vi "Main_UI.vi"() -> ()   [LabVIEW 2012]
uses:
  Donate.ctl
  PortFolio-Provider.ctl
  UI Refs.ctl
  Actions.ctl
  PortFolio/Portfolio.lvclass/Portfolio.ctl
  <vilib>/Utility/miscctls.llb/LVRowAndColumnTypeDef.ctl
  PortFolio/Find_Exchanges.ctl
  PortFolio/Portfolio.lvclass
  Operations/Operations.lvclass
  Exchanges/Exchanges.lvclass
panel:
  in  "Donate":T1
  out "calc Done ?":bool
  out "Current Portfolio Path":path
  out "Version":string="XLPortFolio"
  out "Config File Path":path
  out "Libelles File Path":path
  in  "Search Stock":bool
  in  "Help":bool
  in  "Save":bool
  in  "Print":bool
  in  "Collapse Left":bool
  in  "TabControl":T2(tab)
  out "Performance sur 1an :":sgl format="%.2f%"
  out "% cash":sgl format="%.2f%"
  out "% investi":sgl format="%.2f%"
  out "Montant investi :":sgl format="%.2f€"
  out "Performance Totale :":sgl format="%.2f%"
  out "Investissement total :":sgl format="%.2f€"
  out "Solde Liquidation :":sgl format="%.2f€"
  out "Valeur veille :":sgl format="%.2f€"
  out "Solde espèces :":sgl format="%.2f€"
  out "Evaluation totale :":dbl format="%.2f€"
  in  "Portefeuille":i32(listbox)
  in  "Mettre a jour les cours":bool
  in  "Delete Exch":bool
  in  "Edit Exch":bool
  in  "Add Exch":bool
  in  "Exchanges":i32[](listbox)
  in  "Operations":i32[](listbox)
  in  "Add OP":bool
  in  "Edit OP":bool
  in  "Delete OP":bool
  out "Waveform Graph":waveform(dbl)[](graph)
  in  "Update Hist":bool
  out "Tarifs":waveform(dbl)[](graph) caption="Tarifs des portails Bourses 2017 (en % de Frais)"
  in  "Provider":T3
  out "Table Control 2":string[][](table)=[["12/31/1903 6:00:00 PM", "-0.052"], ["12/31/1903 6:00:00 PM", "-0.133"], ["12/31/1903 6:00:00 PM", "0.097"], ["12/31/1903 6:00:00 PM", "0.043"], ["12/31/1903 6:00:00 PM", "0.408"], ["12/31/1903 6:00:00 PM", "0.144"], ["12/31/1903 6:00:00 PM", "0.183"], ["12/31/1903 6:00:00 PM", "0.589"], ["12/31/1903 6:00:00 PM", "0.287"], ["12/31/1903 6:00:00 PM", "0.424"], ["12/31/1903 6:00:00 PM", "0.399"], ["12/31/1903 6:00:00 PM", "0.495"], ["12/31/1903 6:00:00 PM", "0.848"], ["12/31/1903 6:00:00 PM", "0.550"], ["12/31/1903 6:00:00 PM", "0.762"], ["12/31/1903 6:00:00 PM", "0.686"], ["12/31/1903 6:00:00 PM", "0.766"], ["12/31/1903 6:00:00 PM", "0.760"], ["12/31/1903 6:00:00 PM", "0.913"], ["12/31/1903 6:00:00 PM", "0.929"], ["12/31/1903 6:00:00 PM", "0.800"], ["12/31/1903 6:00:00 PM", "0.958"], ["12/31/1903 6:00:00 PM", "1.034"], ["12/31/1903 6:00:00 PM", "1.183"], ["12/31/1903 6:00:00 PM", "1.132"], ["12/31/1903 6:00:00 PM", "1.155"], ["12/31/1903 6:00:00 PM", "0.931"], ["12/31/1903 6:00:00 PM", "1.036"], ["12/31/1903 6:00:00 PM", "0.780"], ["12/31/1903 6:00:00 PM", "0.999"], ["12/31/1903 6:00:00 PM", "0.907"], ["12/31/1903 6:00:00 PM", "0.915"], ["12/31/1903 6:00:00 PM", "0.726"], ["12/31/1903 6:00:00 PM", "0.758"], ["12/31/1903 6:00:00 PM", "0.769"], ["12/31/1903 6:00:00 PM", "0.879"], ["12/31/1903 6:00:00 PM", "0.573"], ["12/31/1903 6:00:00 PM", "0.830"], ["12/31/1903 6:00:00 PM", "0.796"], ["12/31/1903 6:00:00 PM", "0.546"], ["12/31/1903 6:00:00 PM", "0.413"], ["12/31/1903 6:00:00 PM", "0.602"], ["12/31/1903 6:00:00 PM", "0.547"], ["12/31/1903 6:00:00 PM", "0.573"], ["12/31/1903 6:00:00 PM", "0.326"], ["12/31/1903 6:00:00 PM", "0.432"], ["12/31/1903 6:00:00 PM", "0.132"], ["12/31/1903 6:00:00 PM", "0.157"], ["12/31/1903 6:00:00 PM", "0.194"], ["12/31/1903 6:00:00 PM", "-0.046"], ["12/31/1903 6:00:00 PM", "-0.219"], ["12/31/1903 6:00:00 PM", "-0.209"], ["12/31/1903 6:00:00 PM", "0.007"], ["12/31/1903 6:00:00 PM", "-0.095"], ["12/31/1903 6:00:00 PM", "-0.433"], ["12/31/1903 6:00:00 PM", "-0.258"], ["12/31/1903 6:00:00 PM", "-0.357"], ["12/31/1903 6:00:00 PM", "-0.548"], ["12/31/1903 6:00:00 PM", "-0.712"], ["12/31/1903 6:00:00 PM", "-0.686"], ["12/31/1903 6:00:00 PM", "-0.709"], ["12/31/1903 6:00:00 PM", "-0.790"], ["12/31/1903 6:00:00 PM", "-0.635"], ["12/31/1903 6:00:00 PM", "-0.851"], ["12/31/1903 6:00:00 PM", "-0.953"], ["12/31/1903 6:00:00 PM", "-0.886"], ["12/31/1903 6:00:00 PM", "-0.810"], ["12/31/1903 6:00:00 PM", "-0.966"], ["12/31/1903 6:00:00 PM", "-0.804"], ["12/31/1903 6:00:00 PM", "-1.056"], ["12/31/1903 6:00:00 PM", "-1.070"], ["12/31/1903 6:00:00 PM", "-1.027"], ["12/31/1903 6:00:00 PM", "-0.951"], ["12/31/1903 6:00:00 PM", "-0.862"], ["12/31/1903 6:00:00 PM", "-0.844"], ["12/31/1903 6:00:00 PM", "-1.160"], ["12/31/1903 6:00:00 PM", "-0.880"], ["12/31/1903 6:00:00 PM", "-0.949"], ["12/31/1903 6:00:00 PM", "-1.011"], ["12/31/1903 6:00:00 PM", "-0.802"], ["12/31/1903 6:00:00 PM", "-0.767"], ["12/31/1903 6:00:00 PM", "-0.893"], ["12/31/1903 6:00:00 PM", "-0.788"], ["12/31/1903 6:00:00 PM", "-0.897"], ["12/31/1903 6:00:00 PM", "-0.635"], ["12/31/1903 6:00:00 PM", "-0.592"], ["12/31/1903 6:00:00 PM", "-0.541"], ["12/31/1903 6:00:00 PM", "-0.574"], ["12/31/1903 6:00:00 PM", "-0.511"], ["12/31/1903 6:00:00 PM", "-0.541"], ["12/31/1903 6:00:00 PM", "-0.648"], ["12/31/1903 6:00:00 PM", "-0.499"], ["12/31/1903 6:00:00 PM", "-0.624"], ["12/31/1903 6:00:00 PM", "-0.271"], ["12/31/1903 6:00:00 PM", "-0.120"], ["12/31/1903 6:00:00 PM", "-0.199"], ["12/31/1903 6:00:00 PM", "-0.335"], ["12/31/1903 6:00:00 PM", "-0.056"], ["12/31/1903 6:00:00 PM", "-0.195"], ["12/31/1903 6:00:00 PM", "-0.065"]]
  in  "Collapse Right":bool
  out "Table Control":string[][](table)=[["12/31/1903 6:00:00 PM", "-0.052"], ["12/31/1903 6:00:00 PM", "-0.133"], ["12/31/1903 6:00:00 PM", "0.097"], ["12/31/1903 6:00:00 PM", "0.043"], ["12/31/1903 6:00:00 PM", "0.408"], ["12/31/1903 6:00:00 PM", "0.144"], ["12/31/1903 6:00:00 PM", "0.183"], ["12/31/1903 6:00:00 PM", "0.589"], ["12/31/1903 6:00:00 PM", "0.287"], ["12/31/1903 6:00:00 PM", "0.424"], ["12/31/1903 6:00:00 PM", "0.399"], ["12/31/1903 6:00:00 PM", "0.495"], ["12/31/1903 6:00:00 PM", "0.848"], ["12/31/1903 6:00:00 PM", "0.550"], ["12/31/1903 6:00:00 PM", "0.762"], ["12/31/1903 6:00:00 PM", "0.686"], ["12/31/1903 6:00:00 PM", "0.766"], ["12/31/1903 6:00:00 PM", "0.760"], ["12/31/1903 6:00:00 PM", "0.913"], ["12/31/1903 6:00:00 PM", "0.929"], ["12/31/1903 6:00:00 PM", "0.800"], ["12/31/1903 6:00:00 PM", "0.958"], ["12/31/1903 6:00:00 PM", "1.034"], ["12/31/1903 6:00:00 PM", "1.183"], ["12/31/1903 6:00:00 PM", "1.132"], ["12/31/1903 6:00:00 PM", "1.155"], ["12/31/1903 6:00:00 PM", "0.931"], ["12/31/1903 6:00:00 PM", "1.036"], ["12/31/1903 6:00:00 PM", "0.780"], ["12/31/1903 6:00:00 PM", "0.999"], ["12/31/1903 6:00:00 PM", "0.907"], ["12/31/1903 6:00:00 PM", "0.915"], ["12/31/1903 6:00:00 PM", "0.726"], ["12/31/1903 6:00:00 PM", "0.758"], ["12/31/1903 6:00:00 PM", "0.769"], ["12/31/1903 6:00:00 PM", "0.879"], ["12/31/1903 6:00:00 PM", "0.573"], ["12/31/1903 6:00:00 PM", "0.830"], ["12/31/1903 6:00:00 PM", "0.796"], ["12/31/1903 6:00:00 PM", "0.546"], ["12/31/1903 6:00:00 PM", "0.413"], ["12/31/1903 6:00:00 PM", "0.602"], ["12/31/1903 6:00:00 PM", "0.547"], ["12/31/1903 6:00:00 PM", "0.573"], ["12/31/1903 6:00:00 PM", "0.326"], ["12/31/1903 6:00:00 PM", "0.432"], ["12/31/1903 6:00:00 PM", "0.132"], ["12/31/1903 6:00:00 PM", "0.157"], ["12/31/1903 6:00:00 PM", "0.194"], ["12/31/1903 6:00:00 PM", "-0.046"], ["12/31/1903 6:00:00 PM", "-0.219"], ["12/31/1903 6:00:00 PM", "-0.209"], ["12/31/1903 6:00:00 PM", "0.007"], ["12/31/1903 6:00:00 PM", "-0.095"], ["12/31/1903 6:00:00 PM", "-0.433"], ["12/31/1903 6:00:00 PM", "-0.258"], ["12/31/1903 6:00:00 PM", "-0.357"], ["12/31/1903 6:00:00 PM", "-0.548"], ["12/31/1903 6:00:00 PM", "-0.712"], ["12/31/1903 6:00:00 PM", "-0.686"], ["12/31/1903 6:00:00 PM", "-0.709"], ["12/31/1903 6:00:00 PM", "-0.790"], ["12/31/1903 6:00:00 PM", "-0.635"], ["12/31/1903 6:00:00 PM", "-0.851"], ["12/31/1903 6:00:00 PM", "-0.953"], ["12/31/1903 6:00:00 PM", "-0.886"], ["12/31/1903 6:00:00 PM", "-0.810"], ["12/31/1903 6:00:00 PM", "-0.966"], ["12/31/1903 6:00:00 PM", "-0.804"], ["12/31/1903 6:00:00 PM", "-1.056"], ["12/31/1903 6:00:00 PM", "-1.070"], ["12/31/1903 6:00:00 PM", "-1.027"], ["12/31/1903 6:00:00 PM", "-0.951"], ["12/31/1903 6:00:00 PM", "-0.862"], ["12/31/1903 6:00:00 PM", "-0.844"], ["12/31/1903 6:00:00 PM", "-1.160"], ["12/31/1903 6:00:00 PM", "-0.880"], ["12/31/1903 6:00:00 PM", "-0.949"], ["12/31/1903 6:00:00 PM", "-1.011"], ["12/31/1903 6:00:00 PM", "-0.802"], ["12/31/1903 6:00:00 PM", "-0.767"], ["12/31/1903 6:00:00 PM", "-0.893"], ["12/31/1903 6:00:00 PM", "-0.788"], ["12/31/1903 6:00:00 PM", "-0.897"], ["12/31/1903 6:00:00 PM", "-0.635"], ["12/31/1903 6:00:00 PM", "-0.592"], ["12/31/1903 6:00:00 PM", "-0.541"], ["12/31/1903 6:00:00 PM", "-0.574"], ["12/31/1903 6:00:00 PM", "-0.511"], ["12/31/1903 6:00:00 PM", "-0.541"], ["12/31/1903 6:00:00 PM", "-0.648"], ["12/31/1903 6:00:00 PM", "-0.499"], ["12/31/1903 6:00:00 PM", "-0.624"], ["12/31/1903 6:00:00 PM", "-0.271"], ["12/31/1903 6:00:00 PM", "-0.120"], ["12/31/1903 6:00:00 PM", "-0.199"], ["12/31/1903 6:00:00 PM", "-0.335"], ["12/31/1903 6:00:00 PM", "-0.056"], ["12/31/1903 6:00:00 PM", "-0.195"], ["12/31/1903 6:00:00 PM", "-0.065"]]
  in  "Cancel":bool
  out "Progress Bar":u8(slide) scale=0.0..100.0
  out "Status Bar Text":string="This is the status bar!"
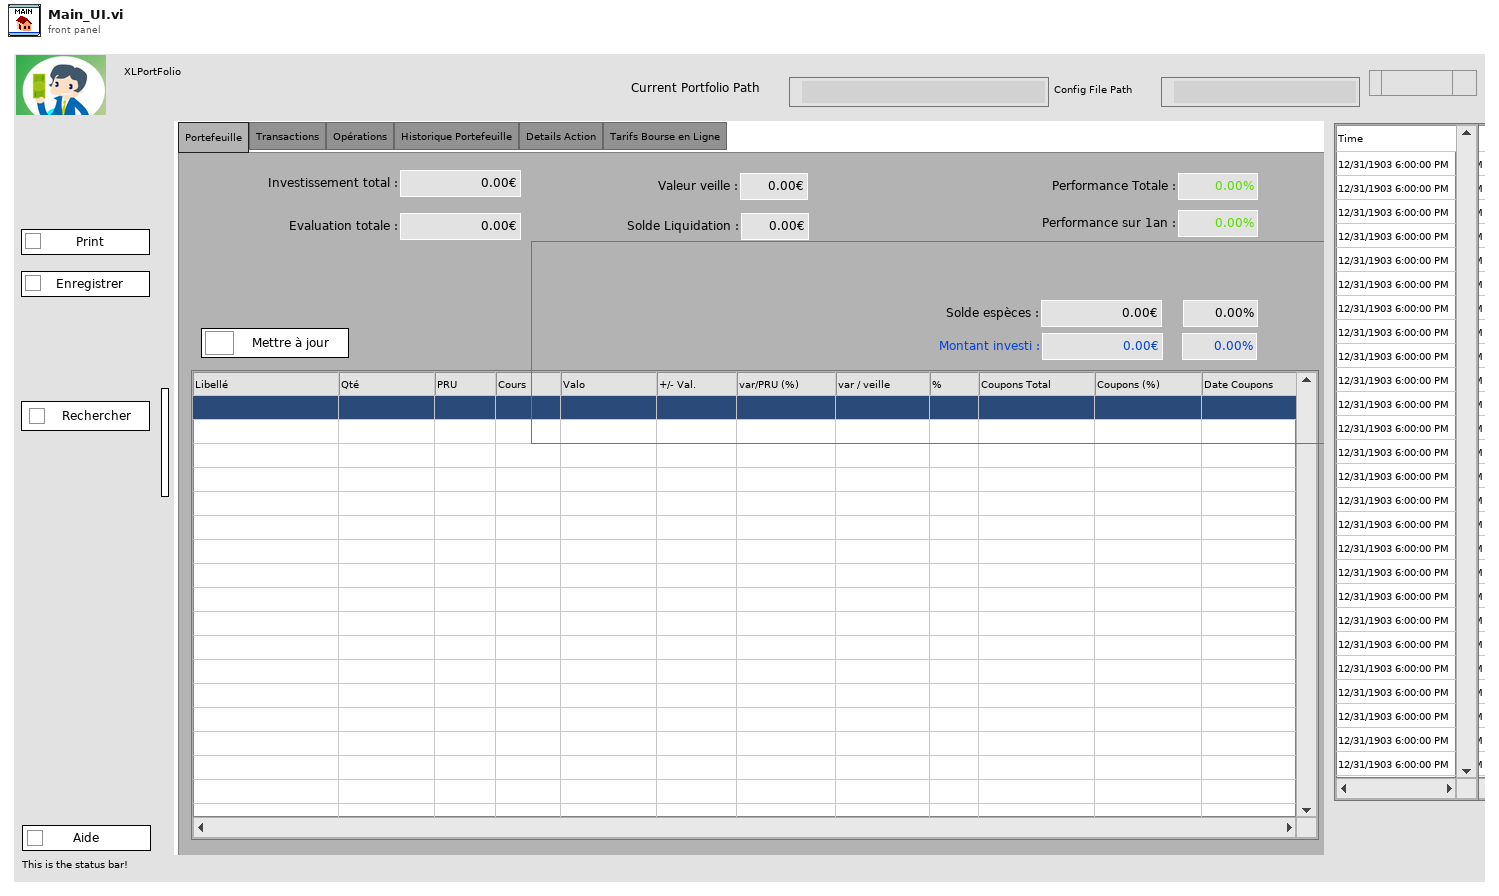
[diagram p1: front panel]
types:
  T1 = typedef "Donate.ctl" = bool
  T2 = enum32{"Portefeuille", "Transactions", "Opérations", "Historique Portefeuille", "Details Action", "Tarifs Bourse en Ligne"}
  T3 = typedef "PortFolio-Provider.ctl" = enum16{"Bourse Direct", "Binck classique", "Boursorama Découverte", "Boursorama Classique", "Boursorama Trader", "Boursorama Ultimate Trader", "IG Actions Euro"}
  T4 = cluster{"Select Printer":string, "Limit number of pages":dbl, "Filename":path, "Prompt for file path":bool, "When saving multiple files":enum32{"Radio Selection 1", "Radio Selection 2"}}
  T5 = enum32{"Portefeuille", "Transactions", "Opérations", "Historique Portefeuille"}
  T6 = typedef "UI Refs.ctl" = cluster{"Cancel Button Ref":refnum<vi>, "Status Bar Text Ref":refnum<vi>, "Progress Bar Ref":refnum<vi>, "This VI":refnum<vi>}
  T7 = typedef "Actions.ctl" = enum16{"Calc", "Calc History", "Test Progress Bar", "Help", "Panel Resize", "Print", "Donate", "Acquire", "Save Portfolio", "New Portfolio", "Open Portfolio", "Add Operation", "Edit Operation", "Delete Operation", "Add Exchange", "Edit Exchange", "Update Operations", "Update Exchanges", "Delete Exchange", "Display tarif", "Update PFLine ToolStrip"}
  T8 = enum8{"Enabled", "Disabled", "Disabled and Grayed Out"}
  T9 = cluster{"FileVersion":string, "FileMajorPart":i32, "FileMinorPart":i32, "FileBuildPart":i32, "FilePrivatePart":i32, "Language":string, "LegalCopyright":string, "FileDescription":string, "CompanyName":string, "ProductName":string, "InternalName":string}
  T10 = typedef "LVRowAndColumnTypeDef.ctl" = cluster{"Row":i32, "Column":i32}
  T11 = typedef "Find_Exchanges.ctl" = enum16{"Find_From_Label", "Find_From_ISIN"}
  T12 = typedef "Portfolio Parameters.ctl" = cluster{"Date":timestamp, "Name":string, "Cash":dbl, "Total":dbl, "Investissements":dbl, "Performance Totale (en %)":dbl, "Performance sur 1 an (en %)":dbl}
  T13 = typedef "Operation Parameters.ctl" = cluster{"Date":timestamp, "Operation Type":T14, "Amount":dbl, "Comment":string, "Currency":T15}
  T14 = typedef "Operation Type Enum.ctl" = enum16{"Coupons", "Dépot", "Retrait", "Intérêts", "Taxe"}
  T15 = typedef "Currencies.ctl" = enum16{"Euro", "Dollar", "Yen", "RIM", "CHF"}
  T16 = typedef "Exchange Parameters.ctl" = cluster{"Date":timestamp, "Exchange Type":T17, "ISIN":string, "Label":string, "Price":dbl, "Qty":dbl, "Currency":T15, "Tax":dbl, "Comment":string, "PRU":dbl}
  T17 = typedef "Exchange.lvclass/Exchange Type Enum.ctl" = enum16{"ACHAT", "VENTE"}
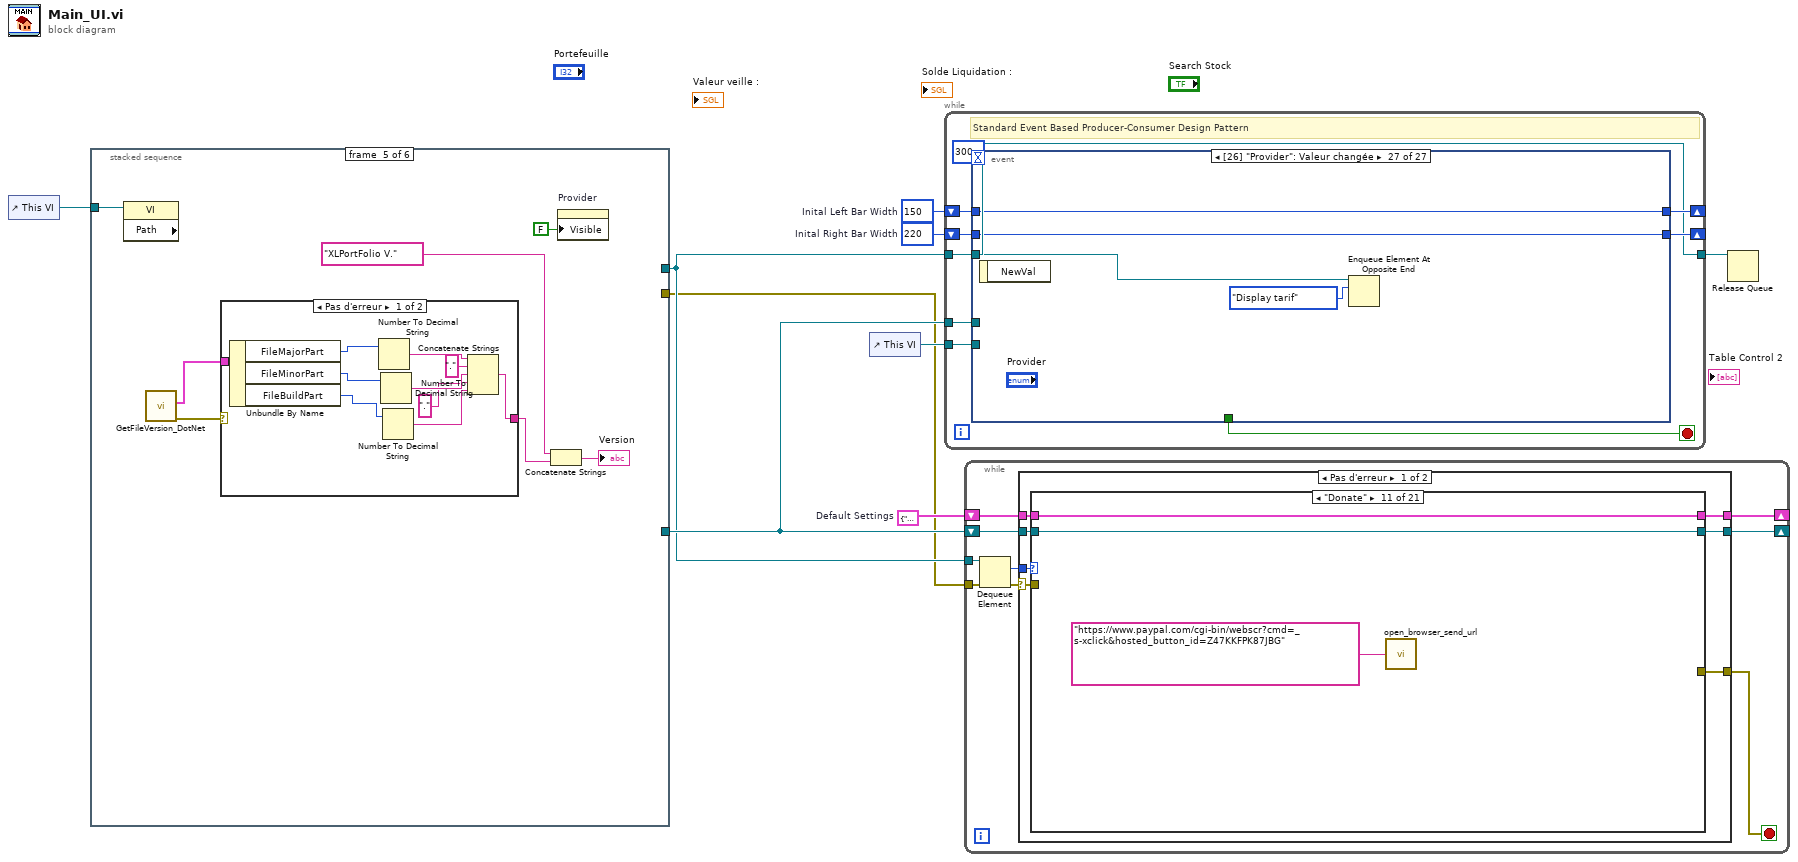
[diagram p0: block diagram]
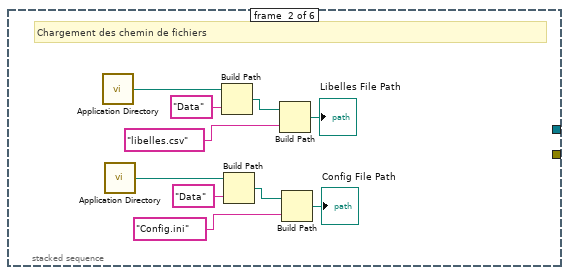
[diagram p3: hidden frame]
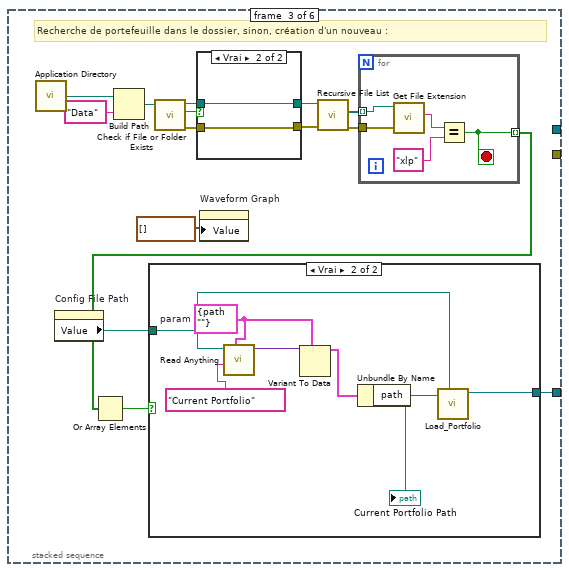
[diagram p4: hidden frame]
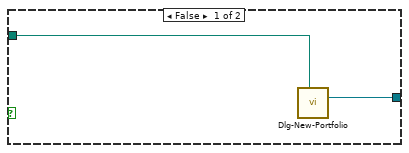
[diagram p5: hidden frame]
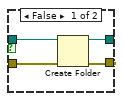
[diagram p6: hidden frame]
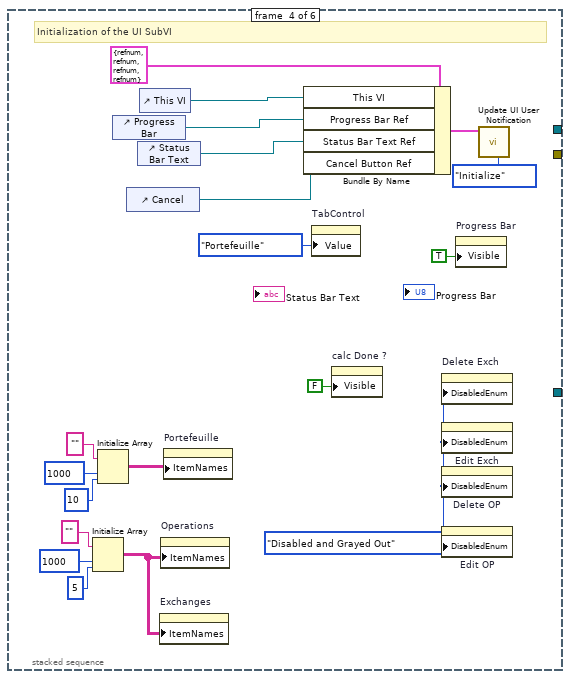
[diagram p7: hidden frame]
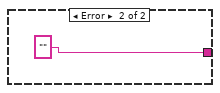
[diagram p8: hidden frame]
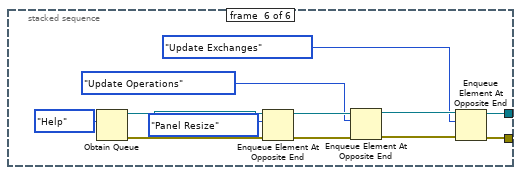
[diagram p9: hidden frame]
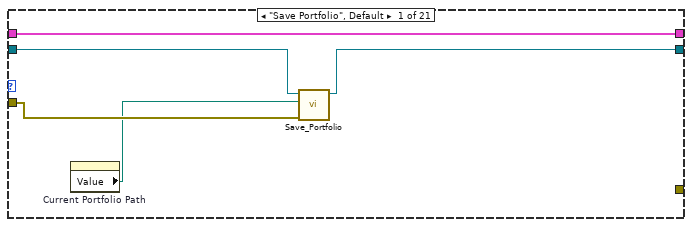
[diagram p10: hidden frame]
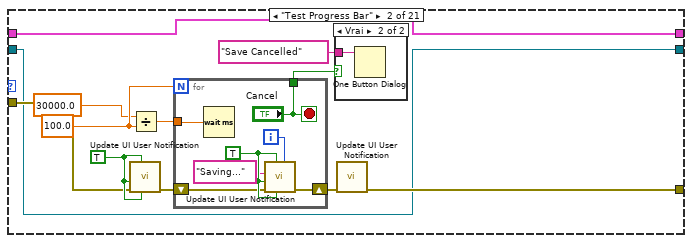
[diagram p11: hidden frame]
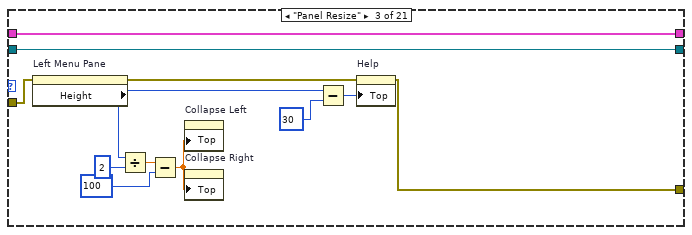
[diagram p13: hidden frame]
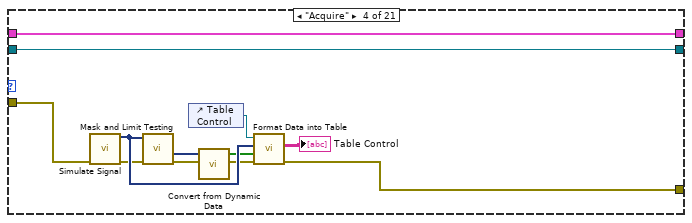
[diagram p14: hidden frame]
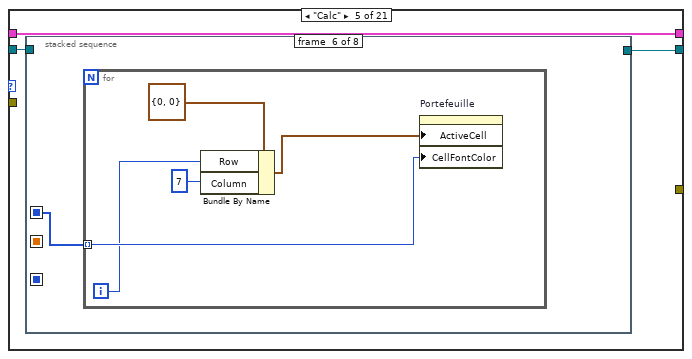
[diagram p15: hidden frame]
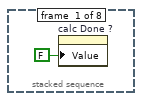
[diagram p16: hidden frame]
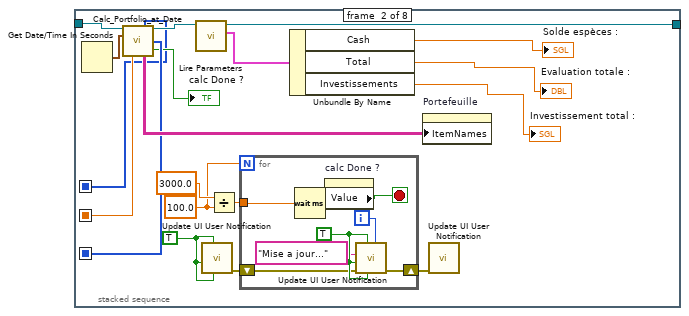
[diagram p17: hidden frame]
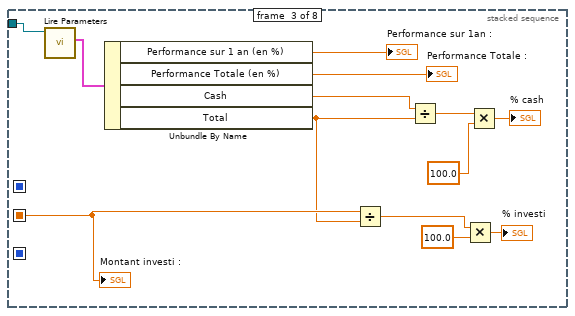
[diagram p18: hidden frame]
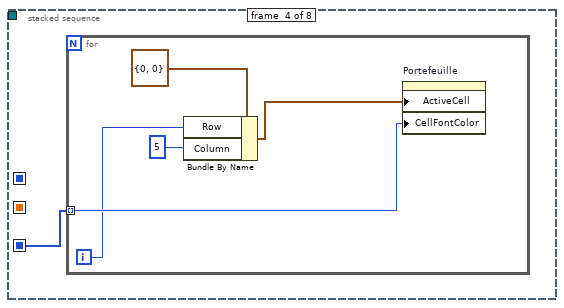
[diagram p19: hidden frame]
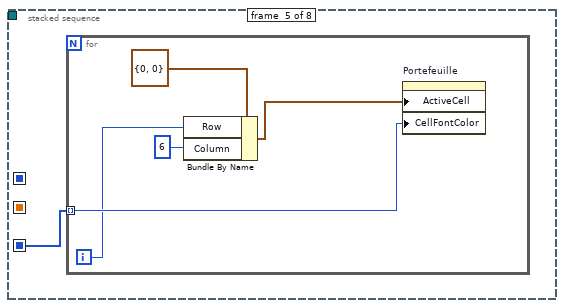
[diagram p20: hidden frame]
diagram:
  w5 = T4 {"Select Printer"="Lab Printer 1", "Limit number of pages"=3.0, "Filename"=path "", "Prompt for file path"=FALSE, "When saving multiple files"=enum."Radio Selection 1"}  # Default Settings
  w8 = 220  # Inital Right Bar Width
  w9 = 150  # Inital Left Bar Width
  n1 = control-ref of="This VI"() -> (w1:refnum<vi>)
  n2 = stacked-sequence {
    tunnel: [_ _ _ _ _ w94] -> w2
    tunnel: [_ _ w34 _ _ _] -> w4
    tunnel: [_ _ _ _ _ w97] -> w3
    tunnel: w1 -> [_ _ _ _ w77 _]
    frame #0 {
    }
    frame #1 {
      # "Chargement des chemin de fichiers"
      n3 = call <vilib>:"Application Directory.vi"() -> ("Application Directory"=w18:path)
      n4 = call <vilib>:"Application Directory.vi"() -> ("Application Directory"=w11:path)
      n5 = Build Path(base path=w18, name or relative path="Data" ("nom ou chemin relatif")) -> (appended path=w16:path)
      n6 = Build Path(base path=w11, name or relative path="Data" ("nom ou chemin relatif")) -> (appended path=w13:path)
      n7 = Build Path(base path=w16, name or relative path="libelles.csv" ("nom ou chemin relatif")) -> (appended path=→"Libelles File Path":path)
      n8 = Build Path(base path=w13, name or relative path="Config.ini" ("nom ou chemin relatif")) -> (appended path=→"Config File Path":path)
    }
    frame #2 {
      # "Recherche de portefeuille dans le dossier, sinon, création d'un nouveau :"
      n9 = call <vilib>:"Application Directory.vi"() -> ("Application Directory"=w33:path)
      n10 = property on="Config File Path" class="Chm"() -> ("Value"=w21:path)  [unwired: 2 in, 2 out]
      n11 = Build Path(base path=w33, name or relative path="Data" ("nom ou chemin relatif")) -> (appended path=w31:path)
      n12 = call <vilib>:"Check if File or Folder Exists.vi"("path"=w31) -> ("error out"=w28:errorcluster, "file or folder exists?"=w30:bool, "dup path"=w29:path)  [unwired: 8 in]
      n13 = case shown="Vrai" w30 {
        tunnel: w29 -> [w52 w53]
        tunnel: w28 -> [w51 w54]
        tunnel: [w50 w54] -> w26
        tunnel: [w49 w53] -> w27
        frame False {
          n14 = Create Folder(path (use dialog)=w52, error in=w51) -> (created path=w49:path, error out=w50:errorcluster)  [unwired: 1 in, 1 out]
        }
        frame True {
        }
      }
      n15 = property on="Waveform Graph" class="GraphWF (strict)"("Value"=waveform(dbl)[] [] ("Waveform Graph")) -> ()  [unwired: 2 in, 2 out]
      n16 = call <vilib>:"Recursive File List.vi"("error in (no error)"=w26, "Folder Path"=w27) -> ("error out"=w24:errorcluster, "All Files in Dir"=w25:path[])  [unwired: 5 in, 3 out]
      n17 = for {
        tunnel: w25 -> [w39] mode=indexing
        tunnel: w24 -> [w38]
        tunnel: [w35] -> w23 mode=indexing
        stop <- w35 stop-if-true
        n18 = call <vilib>:"Get File Extension.vi"("error in (no error)"=w38, "file"=w39) -> ("lowercase file extension"=w37:string)  [unwired: 6 in, 3 out]
        n19 = Equal?(x=w37, y="xlp") -> (x = y?=w35:bool)
      }
      n20 = Or Array Elements(Boolean array=w23) -> (logical OR=w22:bool)
      n21 = case shown="Vrai" w22 {
        tunnel: [w41 w46] -> w34
        tunnel: w21 -> [w40 w45]
        frame False {
          n22 = call "Dlg-New-Portfolio.vi"("Config File Path"=w40) -> ("Portfolio out"=w41:refnum<class "Portfolio.lvclass">)  [unwired: 8 in, 2 out]
        }
        frame True {
          w44 = cluster{"path":path} {"path"=path ""}  # param
          n23 = call "Read Anything.vi"("Type of Anything"=w44, "Section Name (Name of \"Type of Anything\")"="Current Portfolio" ("Section Name (Name of \"Anything\")"), "Path (dialog)"=w45) -> ("Anything"=w48:variant)  [unwired: 6 in, 2 out]
          n24 = Variant To Data(type=w44, Variant=w48) -> (data=w43:cluster{"path":path})  [unwired: 1 in, 1 out]
          n25 = Unbundle By Name(w43) -> ("path"=w42:path)
          "Current Portfolio Path" <- w42
          n26 = call "Load_Portfolio.vi"("Config File path"=w45, "path"=w42) -> ("Portfolio en sortie"=w46:refnum<class "Portfolio.lvclass">)  [unwired: 8 in, 1 out]
        }
      }
    }
    frame #3 {
      w57 = T8."Disabled and Grayed Out" ("Désactivé")
      # "Initialization of the UI SubVI"
      n27 = Initialize Array("", 1000, 5 ("taille de la dimension")) -> (w59:string[][])
      n28 = Initialize Array("", 1000, 10 ("taille de la dimension")) -> (w60:string[][])
      n29 = control-ref of="Progress Bar"() -> (w70:refnum<vi>)
      n30 = control-ref of="Cancel"() -> (w58:refnum<vi>)
      n31 = control-ref of="Status Bar Text"() -> (w69:refnum<vi>)
      n32 = control-ref of="This VI"() -> (w71:refnum<vi>)
      n33 = property on="Exchanges" class="ListeMCol (strict)"("ItemNames"=w59) -> ()  [unwired: 2 in, 2 out]
      n34 = property on="Operations" class="ListeMCol (strict)"("ItemNames"=w59) -> ()  [unwired: 2 in, 2 out]
      n35 = property on="Portefeuille" class="ListeMCol (strict)"("ItemNames"=w60) -> ()  [unwired: 2 in, 2 out]
      n36 = Bundle By Name(cluster=T6 {"Cancel Button Ref"=refnum, "Status Bar Text Ref"=refnum, "Progress Bar Ref"=refnum, "This VI"=refnum} ("UI Refs In"), "This VI"=w71, "Progress Bar Ref"=w70, "Status Bar Text Ref"=w69, "Cancel Button Ref"=w58) -> (w68:T6)
      n37 = property on="TabControl" class="Onglet (strict)"("Value"=T5."Portefeuille" ("TabControl")) -> ()  [unwired: 2 in, 2 out]
      n38 = property on="calc Done ?" class="Bool (strict)"("Visible"=FALSE) -> ()  [unwired: 2 in, 2 out]
      n39 = property on="Delete Exch" class="Bool"("DisabledEnum"=w57) -> ()  [unwired: 2 in, 2 out]
      n40 = property on="Edit Exch" class="Bool"("DisabledEnum"=w57) -> ()  [unwired: 2 in, 2 out]
      n41 = property on="Delete OP" class="Bool"("DisabledEnum"=w57) -> ()  [unwired: 2 in, 2 out]
      n42 = property on="Edit OP" class="Bool"("DisabledEnum"=w57) -> ()  [unwired: 2 in, 2 out]
      n43 = property on="Progress Bar" class="Gliss (strict)"("Visible"=TRUE) -> ()  [unwired: 2 in, 2 out]
      n44 = call "Update UI User Notification.vi"("Action"=enum16{"Reset", "Set", "Initialize"}."Initialize", "UI Refs In"=w68) -> ()  [unwired: 8 in, 2 out]
    }
    frame #4 {
      n45 = property class="VI" props=["Path"](reference=w77) -> ()  [unwired: 1 in, 3 out]
      n46 = call "GetFileVersion_DotNet.vi"() -> ("error out"=w79:errorcluster, "File Info Out"=w78:T9)  [unwired: 9 in, 1 out]
      n47 = case shown="Pas d'erreur" w79 {
        tunnel: [w84 "" ("chaîne")] -> w75
        tunnel: w78 -> [w90 _]
        frame No Error {
          n48 = Unbundle By Name(w90) -> ("FileMajorPart"=w89:i32, "FileMinorPart"=w88:i32, "FileBuildPart"=w83:i32)
          n49 = Number To Decimal String(number=w89) -> (decimal integer string=w86:string)  [unwired: 1 in]
          n50 = Number To Decimal String(number=w88) -> (decimal integer string=w85:string)  [unwired: 1 in]
          n51 = Number To Decimal String(number=w83) -> (decimal integer string=w81:string)  [unwired: 1 in]
          n52 = Concatenate Strings(w86, "." ("chaîne"), w85, "." ("chaîne"), w81) -> (w84:string)
        }
        frame Error {
        }
      }
      n53 = Concatenate Strings("XLPortFolio V." ("chaîne"), w75) -> (→"Version":string)
      n54 = property on="Provider" class="Énum (strict)"("Visible"=FALSE) -> ()  [unwired: 2 in, 2 out]
    }
    frame #5 {
      n55 = Obtain Queue(element data type=Actions."Help" ("Enum")) -> (queue out=w100:refnum<queue>, error out=w102:errorcluster)  [unwired: 4 in, 1 out]
      n56 = Enqueue Element At Opposite End(queue=w100, element=Actions."Panel Resize" ("Enum"), error in (no error)=w102) -> (queue out=w99:refnum<queue>, error out=w98:errorcluster)  [unwired: 1 in, 1 out]
      n57 = Enqueue Element At Opposite End(queue=w99, element=Actions."Update Operations" ("Enum"), error in (no error)=w98) -> (queue out=w96:refnum<queue>, error out=w95:errorcluster)  [unwired: 1 in, 1 out]
      n58 = Enqueue Element At Opposite End(queue=w96, element=Actions."Update Exchanges" ("Enum"), error in (no error)=w95) -> (queue out=w97:refnum<queue>, error out=w94:errorcluster)  [unwired: 1 in, 1 out]
    }
  }
  n59 = control-ref of="This VI"() -> (w7:refnum<vi>)
  n60 = while {
    shift-right: [w109] -> _
    shift-left: w9 -> [w112]
    shift-right: [w108] -> _
    shift-left: w8 -> [w107]
    tunnel: w7 -> [w110]
    tunnel: w3 -> [w106]
    tunnel: [w106] -> w6
    tunnel: w4 -> [w104]
    stop <- w111 stop-if-true
    # "Standard Event Based Producer-Consumer Design Pattern"
    n61 = event shown="[26] \"Provider\": Valeur changée" {
      selector: _ -> [_ _ _ _ _ _ _ _ _ _ _ _ _ _ _ _ _ _ _ _ _ _ _ _ _ _ _]
      dyn-events: _ -> [_ _ _ _ _ _ _ _ _ _ _ _ _ _ _ _ _ _ _ _ _ _ _ _ _ _ _]
      timeout: 300 -> [_ _ _ _ _ _ _ _ _ _ _ _ _ _ _ _ _ _ _ _ _ _ _ _ _ _ _]
      tunnel: w112 -> [w115 w150 w163 w176 w178 w183 w187 w207 w219 w233 w239 w245 w251 w257 w263 w267 w271 w273 w284 w299 w302 w305 w309 w314 w318 w322 w328]
      tunnel: [w115 w150 w163 w176 w178 w183 w187 w207 w219 w233 w239 w245 w251 w257 w263 w267 w271 w274 w285 w299 w302 w305 w309 w314 w318 w322 w328] -> w109
      tunnel: [_ _ _ _ w179 _ _ _ _ _ _ _ _ _ _ _ _ _ _ _ _ _ _ _ _ _ _] -> w111
      tunnel: w110 -> [_ _ _ _ _ _ _ _ _ _ _ _ _ _ _ _ _ _ w283 _ _ _ _ _ _ _ _]
      tunnel: [w114 w149 w162 w175 w177 w182 w186 w206 w218 w232 w238 w244 w250 w256 w262 w266 w270 w272 w280 w298 w301 w304 w308 w313 w317 w321 w327] -> w108
      tunnel: w107 -> [w114 w149 w162 w175 w177 w182 w186 w206 w218 w232 w238 w244 w250 w256 w262 w266 w270 w272 w279 w298 w301 w304 w308 w313 w317 w321 w327]
      tunnel: w106 -> [_ w147 _ _ _ w180 w184 w205 w217 w230 w236 w242 w248 w254 w260 w265 w268 _ _ _ _ w303 w310 w311 w315 w320 w326]
      tunnel: w104 -> [w113 _ w155 w169 _ _ _ _ _ _ _ _ _ _ _ _ _ _ _ _ _ _ _ _ _ _ _]
      event Timeout {
        n62 = event-data() -> ()  [unwired: 1 in, 1 out]
        n63 = stacked-sequence {
          tunnel: w113 -> [w117 _ _]
          frame #0 {
            n64 = call "Lire Operations.vi"("Portfolio en entrée"=w117) -> ("Operations.lvclass"=w128:refnum<class "Operations.lvclass">)  [unwired: 9 in, 1 out]
            n65 = call "Lire Exchanges.vi"("Portfolio en entrée"=w117) -> ("Exchanges.lvclass"=w118:refnum<class "Exchanges.lvclass">)  [unwired: 9 in, 1 out]
            n66 = call "Size Operations.vi"("Operations en entrée"=w128) -> ("size"=w127:i32)  [unwired: 8 in, 2 out]
            n67 = call "Size Exchanges.vi"("Exchanges en entrée"=w118) -> ("size"=w116:i32)  [unwired: 8 in, 2 out]
            n68 = Greater Than 0?(x=w127) -> (x > 0?=w123:bool)
            n69 = Greater Than 0?(x=w116) -> (x > 0?=w122:bool)
            n70 = Select(t=T8."Enabled" ("Désactivé"), s=w123, f=T8."Disabled and Grayed Out" ("Désactivé")) -> (s? t:f=w124:T8)
            n71 = Select(t=T8."Enabled" ("Désactivé"), s=w122, f=T8."Disabled and Grayed Out" ("Désactivé")) -> (s? t:f=w119:T8)
            n72 = property on="Edit OP" class="Bool"("DisabledEnum"=w124) -> ()  [unwired: 2 in, 2 out]
            n73 = property on="Delete OP" class="Bool"("DisabledEnum"=w124) -> ()  [unwired: 2 in, 2 out]
            n74 = property on="Edit Exch" class="Bool"("DisabledEnum"=w119) -> ()  [unwired: 2 in, 2 out]
            n75 = property on="Delete Exch" class="Bool"("DisabledEnum"=w119) -> ()  [unwired: 2 in, 2 out]
          }
          frame #1 {
            n76 = property on="Performance Totale :" class="NumNb (strict)"() -> ("Value"=w129:sgl)  [unwired: 2 in, 2 out]
            n77 = Equal To 0?(x=w129) -> (x = 0?=w131:bool)
            n78 = case shown="Faux" w131 {
              tunnel: [w133 u32 0 ("Color")] -> w130
              tunnel: w129 -> [w136 _]
              frame False {
                n79 = Greater Than 0?(x=w136) -> (x > 0?=w135:bool)
                n80 = Select(t=u32 5823744 ("Color"), s=w135, f=u32 16711680 ("Color")) -> (s? t:f=w133:u32)
              }
              frame True {
              }
            }
            n81 = property on="Performance Totale :" class="NumNb (strict)"("NumText.TextColor"=w130) -> ()  [unwired: 2 in, 2 out]
          }
          frame #2 {
            n82 = property on="Performance sur 1an :" class="NumNb (strict)"() -> ("Value"=w139:sgl)  [unwired: 2 in, 2 out]
            n83 = Equal To 0?(x=w139) -> (x = 0?=w140:bool)
            n84 = case shown="Faux" w140 {
              tunnel: [w142 u32 0 ("Color")] -> w138
              tunnel: w139 -> [w145 _]
              frame False {
                n85 = Greater Than 0?(x=w145) -> (x > 0?=w144:bool)
                n86 = Select(t=u32 5823744 ("Color"), s=w144, f=u32 16711680 ("Color")) -> (s? t:f=w142:u32)
              }
              frame True {
              }
            }
            n87 = property on="Performance sur 1an :" class="NumNb (strict)"("NumText.TextColor"=w138) -> ()  [unwired: 2 in, 2 out]
          }
        }
      }
      event "Update Hist": Value Change {
        n88 = event-data() -> ()  [unwired: 1 in, 1 out]
        n89 = Enqueue Element At Opposite End(queue=w147, element=Actions."Calc History" ("Enum")) -> ()  [unwired: 2 in, 3 out]
      }
      event "Operations": Mouse Up {
        n90 = event-data() -> ()  [unwired: 1 in, 1 out]
        n91 = call "Lire Operations.vi"("Portfolio en entrée"=w155) -> ("Operations.lvclass"=w154:refnum<class "Operations.lvclass">)  [unwired: 9 in, 1 out]
        n92 = call "Size Operations.vi"("Operations en entrée"=w154) -> ("size"=w153:i32)  [unwired: 8 in, 2 out]
        n93 = Index Array(array="Operations") -> (element=w160:i32)  [unwired: 1 in]
        n94 = Greater Or Equal To 0?(x=w160) -> (x >= 0?=w157:bool)
        n95 = Greater Than 0?(x=w153) -> (x > 0?=w152:bool)
        n96 = And(x=w157, y=w152) -> (x .and. y?=w156:bool)
        n97 = Select(t=T8."Enabled" ("Désactivé"), s=w156, f=T8."Disabled and Grayed Out" ("Désactivé")) -> (s? t:f=w151:T8)
        n98 = property on="Edit OP" class="Bool"("DisabledEnum"=w151) -> ()  [unwired: 2 in, 2 out]
        n99 = property on="Delete OP" class="Bool"("DisabledEnum"=w151) -> ()  [unwired: 2 in, 2 out]
      }
      event "Exchanges": Mouse Up {
        n100 = event-data() -> ()  [unwired: 1 in, 1 out]
        n101 = call "Lire Exchanges.vi"("Portfolio en entrée"=w169) -> ("Exchanges.lvclass"=w168:refnum<class "Exchanges.lvclass">)  [unwired: 9 in, 1 out]
        n102 = call "Size Exchanges.vi"("Exchanges en entrée"=w168) -> ("size"=w167:i32)  [unwired: 8 in, 2 out]
        n103 = Index Array(array="Exchanges") -> (element=w174:i32)  [unwired: 1 in]
        n104 = Greater Or Equal To 0?(x=w174) -> (x >= 0?=w171:bool)
        n105 = Greater Than 0?(x=w167) -> (x > 0?=w166:bool)
        n106 = And(x=w171, y=w166) -> (x .and. y?=w170:bool)
        n107 = Select(t=T8."Enabled" ("Désactivé"), s=w170, f=T8."Disabled and Grayed Out" ("Désactivé")) -> (s? t:f=w164:T8)
        n108 = property on="Edit Exch" class="Bool"("DisabledEnum"=w164) -> ()  [unwired: 2 in, 2 out]
        n109 = property on="Delete Exch" class="Bool"("DisabledEnum"=w164) -> ()  [unwired: 2 in, 2 out]
      }
      event Panel Close? {
        w179 = TRUE ("Discard?")
        n110 = event-data() -> ()  [unwired: 1 in, 1 out]
        n111 = event-data("Discard?"=w179) -> ()  [unwired: 1 in, 1 out]
      }
      event "Help": Value Change {
        n112 = event-data() -> ()  [unwired: 1 in, 1 out]
        n113 = Enqueue Element At Opposite End(queue=w180, element=Actions."Help" ("Enum")) -> ()  [unwired: 2 in, 3 out]
      }
      event Menu Selection (User) {
        n114 = event-data() -> ("ItemTag"=w185:string)  [unwired: 1 in, 3 out]
        n115 = case shown="\"Open Portfolio\"" w185 {
          tunnel: w184 -> [_ w189 w191 w197 w199 w201 w203]
          frame "False", Default {
          }
          frame "Help" {
            n116 = Enqueue Element At Opposite End(queue=w189, element=Actions."Help" ("Enum")) -> ()  [unwired: 2 in, 3 out]
          }
          frame "New Portfolio" {
            n117 = Enqueue Element At Opposite End(queue=w191, element=Actions."New Portfolio" ("Enum")) -> ()  [unwired: 2 in, 3 out]
          }
          frame "Open Portfolio" {
            n118 = Enqueue Element At Opposite End(queue=w197, element=Actions."Open Portfolio" ("Enum")) -> (queue out=w195:refnum<queue>)  [unwired: 2 in, 2 out]
            n119 = Enqueue Element At Opposite End(queue=w195, element=Actions."Update Operations" ("Enum")) -> (queue out=w194:refnum<queue>)  [unwired: 2 in, 2 out]
            n120 = Enqueue Element At Opposite End(queue=w194, element=Actions."Update Exchanges" ("Enum")) -> ()  [unwired: 2 in, 3 out]
          }
          frame "Settings" {
            n121 = Enqueue Element At Opposite End(queue=w199, element=Actions."Donate" ("Enum")) -> ()  [unwired: 2 in, 3 out]
          }
          frame "Print" {
            n122 = Enqueue Element At Opposite End(queue=w201, element=Actions."Print" ("Enum")) -> ()  [unwired: 2 in, 3 out]
          }
          frame "Save Portfolio" {
            n123 = Enqueue Element At Opposite End(queue=w203, element=Actions."Save Portfolio" ("Enum")) -> ()  [unwired: 2 in, 3 out]
          }
        }
      }
      event "Operations": Shortcut Menu Selection (User) {
        n124 = event-data() -> ("ItemTag"=w204:string)  [unwired: 1 in]
        n125 = case shown="\"OP_EDIT\"" w204 {
          tunnel: w205 -> [_ w211 w215]
          frame "False", Default {
          }
          frame "OP_EDIT" {
            n126 = Enqueue Element At Opposite End(queue=w211, element=Actions."Edit Operation" ("Enum")) -> (queue out=w209:refnum<queue>)  [unwired: 2 in, 2 out]
            n127 = Enqueue Element At Opposite End(queue=w209, element=Actions."Update Operations" ("Enum")) -> ()  [unwired: 2 in, 3 out]
          }
          frame "OP_DEL" {
            n128 = Enqueue Element At Opposite End(queue=w215, element=Actions."Delete Operation" ("Enum")) -> (queue out=w213:refnum<queue>)  [unwired: 2 in, 2 out]
            n129 = Enqueue Element At Opposite End(queue=w213, element=Actions."Update Operations" ("Enum")) -> ()  [unwired: 2 in, 3 out]
          }
        }
      }
      event "Exchanges": Shortcut Menu Selection (User) {
        n130 = event-data() -> ("ItemTag"=w216:string)  [unwired: 1 in]
        n131 = case shown="\"EXCH_EDIT\"" w216 {
          tunnel: w217 -> [_ w223 w227]
          frame "False", Default {
          }
          frame "EXCH_EDIT" {
            n132 = Enqueue Element At Opposite End(queue=w223, element=Actions."Edit Exchange" ("Enum")) -> (queue out=w221:refnum<queue>)  [unwired: 2 in, 2 out]
            n133 = Enqueue Element At Opposite End(queue=w221, element=Actions."Update Exchanges" ("Enum")) -> ()  [unwired: 2 in, 3 out]
          }
          frame "EXCH_DEL" {
            n134 = Enqueue Element At Opposite End(queue=w227, element=Actions."Delete Exchange" ("Enum")) -> (queue out=w225:refnum<queue>)  [unwired: 2 in, 2 out]
            n135 = Enqueue Element At Opposite End(queue=w225, element=Actions."Update Exchanges" ("Enum")) -> ()  [unwired: 2 in, 3 out]
          }
        }
      }
      event "Add OP": Value Change {
        n136 = event-data() -> ()  [unwired: 1 in, 1 out]
        n137 = Enqueue Element At Opposite End(queue=w230, element=Actions."Add Operation" ("Enum")) -> (queue out=w229:refnum<queue>)  [unwired: 2 in, 2 out]
        n138 = Enqueue Element At Opposite End(queue=w229, element=Actions."Update Operations" ("Enum")) -> ()  [unwired: 2 in, 3 out]
      }
      event "Add Exch": Value Change {
        n139 = event-data() -> ()  [unwired: 1 in, 1 out]
        n140 = Enqueue Element At Opposite End(queue=w236, element=Actions."Add Exchange" ("Enum")) -> (queue out=w235:refnum<queue>)  [unwired: 2 in, 2 out]
        n141 = Enqueue Element At Opposite End(queue=w235, element=Actions."Update Exchanges" ("Enum")) -> ()  [unwired: 2 in, 3 out]
      }
      event "Edit OP": Value Change {
        n142 = event-data() -> ()  [unwired: 1 in, 1 out]
        n143 = Enqueue Element At Opposite End(queue=w242, element=Actions."Edit Operation" ("Enum")) -> (queue out=w240:refnum<queue>)  [unwired: 2 in, 2 out]
        n144 = Enqueue Element At Opposite End(queue=w240, element=Actions."Update Operations" ("Enum")) -> ()  [unwired: 2 in, 3 out]
      }
      event "Edit Exch": Value Change {
        n145 = event-data() -> ()  [unwired: 1 in, 1 out]
        n146 = Enqueue Element At Opposite End(queue=w248, element=Actions."Edit Exchange" ("Enum")) -> (queue out=w246:refnum<queue>)  [unwired: 2 in, 2 out]
        n147 = Enqueue Element At Opposite End(queue=w246, element=Actions."Update Exchanges" ("Enum")) -> ()  [unwired: 2 in, 3 out]
      }
      event "Delete OP": Value Change {
        n148 = event-data() -> ()  [unwired: 1 in, 1 out]
        n149 = Enqueue Element At Opposite End(queue=w254, element=Actions."Delete Operation" ("Enum")) -> (queue out=w253:refnum<queue>)  [unwired: 2 in, 2 out]
        n150 = Enqueue Element At Opposite End(queue=w253, element=Actions."Update Operations" ("Enum")) -> ()  [unwired: 2 in, 3 out]
      }
      event "Delete Exch": Value Change {
        n151 = event-data() -> ()  [unwired: 1 in, 1 out]
        n152 = Enqueue Element At Opposite End(queue=w260, element=Actions."Delete Exchange" ("Enum")) -> (queue out=w259:refnum<queue>)  [unwired: 2 in, 2 out]
        n153 = Enqueue Element At Opposite End(queue=w259, element=Actions."Update Exchanges" ("Enum")) -> ()  [unwired: 2 in, 3 out]
      }
      event Panel Resize {
        n154 = event-data() -> ()  [unwired: 1 in, 1 out]
        n155 = Enqueue Element At Opposite End(queue=w265, element=Actions."Panel Resize" ("Enum")) -> ()  [unwired: 2 in, 3 out]
      }
      event "Print": Value Change {
        n156 = event-data() -> ()  [unwired: 1 in, 3 out]
        n157 = Enqueue Element At Opposite End(queue=w268, element=Actions."Print" ("Enum")) -> ()  [unwired: 2 in, 3 out]
      }
      event "Collapse Left": Value Change {
        n158 = event-data() -> ("NewVal"=w275:bool)  [unwired: 1 in]
        n159 = case shown="Faux" w275 {
          tunnel: [w276 w277] -> w274
          tunnel: w273 -> [w276 _]
          frame False {
            n160 = property on="Left Bar Splitter" class="BarreDiv"("Position"=w276) -> ()  [unwired: 2 in, 2 out]
          }
          frame True {
            n161 = property on="Left Bar Splitter" class="BarreDiv"("Position"=6 ("Splitter Position")) -> ("Position"=w277:i32)  [unwired: 2 in, 2 out]
          }
        }
      }
      event "Collapse Right": Value Change {
        n162 = event-data() -> ("NewVal"=w286:bool)  [unwired: 1 in]
        n163 = property class="VI"(reference=w283) -> ("Panel"=w282:refnum<vi>)  [unwired: 1 in, 2 out]
        n164 = property class="FA"(reference=w282) -> ("Width"=w281:u32)  [unwired: 1 in, 2 out]
        n165 = case shown="Vrai" w286 {
          tunnel: [w290 w294] -> w285
          tunnel: w284 -> [w290 w294]
          tunnel: w281 -> [w288 w292]
          tunnel: [w287 w291] -> w280
          tunnel: w279 -> [w287 _]
          frame False {
            n166 = Subtract(x=w288, y=w287) -> (x-y=w289:u32)
            n167 = property on="Right Bar Splitter" class="BarreDiv"("Position"=w289) -> ()  [unwired: 2 in, 2 out]
          }
          frame True {
            n168 = Subtract(x=w292, y=16 ("Splitter Position")) -> (x-y=w295:u32)
            n169 = property on="Right Bar Splitter" class="BarreDiv"("Position"=w295) -> ("Position"=w293:i32)  [unwired: 2 in, 2 out]
            n170 = Subtract(x=w292, y=w293) -> (x-y=w291:u32)
          }
        }
      }
      event "Help", "Save", "Print": Mouse Enter {
        n171 = event-data() -> ("CtlRef"=w300:refnum<vi>)  [unwired: 1 in]
        n172 = property class="Bool"(reference=w300) -> ("TipStrip"=w297:string)  [unwired: 1 in, 2 out]
        n173 = call "Update UI User Notification.vi"("Status Bar (\"\")"=w297) -> ()  [unwired: 9 in, 2 out]
      }
      event "Help", "Save", "Print": Mouse Leave {
        # "The mouse left a mouseover item, reset the status bar"
        n174 = event-data() -> ()  [unwired: 1 in, 1 out]
        n175 = call "Update UI User Notification.vi"() -> ()  [unwired: 10 in, 2 out]
      }
      event Value Change {
        n176 = event-data() -> ()  [unwired: 1 in, 1 out]
        n177 = Enqueue Element At Opposite End(queue=w303, element=Actions."Donate" ("Enum")) -> ()  [unwired: 2 in, 3 out]
      }
      event "Save": Value Change {
        n178 = event-data() -> ()  [unwired: 1 in, 1 out]
        n179 = Enqueue Element At Opposite End(queue=w310, element=Actions."Save Portfolio" ("Enum")) -> ()  [unwired: 2 in, 3 out]
      }
      event "Mettre a jour les cours": Value Change {
        n180 = event-data() -> ()  [unwired: 1 in, 1 out]
        n181 = Enqueue Element At Opposite End(queue=w311, element=Actions."Calc" ("Enum")) -> ()  [unwired: 2 in, 3 out]
      }
      event "Portefeuille": Value Change {
        n182 = event-data() -> ()  [unwired: 1 in, 1 out]
        n183 = Enqueue Element At Opposite End(queue=w315, element=Actions."Update PFLine ToolStrip" ("Enum")) -> ()  [unwired: 2 in, 3 out]
      }
      event "TabControl": Value Change {
        n184 = event-data() -> ("NewVal"=w319:T2)  [unwired: 1 in]
        n185 = case shown="\"Tarifs Bourse en Ligne\"" w319 {
          tunnel: w320 -> [_ w323]
          frame "Portefeuille", Default {
          }
          frame "Tarifs Bourse en Ligne" {
            n186 = Enqueue Element At Opposite End(queue=w323, element=Actions."Display tarif" ("Enum")) -> ()  [unwired: 2 in, 3 out]
          }
        }
      }
      event Value Change {
        n187 = event-data() -> ()  [unwired: 1 in, 1 out]
        n188 = Enqueue Element At Opposite End(queue=w326, element=Actions."Display tarif" ("Enum")) -> ()  [unwired: 2 in, 3 out]
      }
    }
  }
  n189 = while {
    tunnel: w3 -> [w337]
    tunnel: w2 -> [w333]
    shift-right: [w332] -> _
    shift-left: w5 -> [w331]
    shift-right: [w329] -> _
    shift-left: w4 -> [w330]
    stop <- w334 stop-if-true
    n190 = Dequeue Element(queue=w337, error in (no error)=w333) -> (element=w335:T7, error out=w336:errorcluster)  [unwired: 1 in, 2 out]
    n191 = case shown="Pas d'erreur" w336 {
      selector: w336 -> [w343 w642]
      tunnel: w335 -> [w344 _]
      tunnel: [w342 w642] -> w334
      tunnel: [w338 w641] -> w332
      tunnel: w331 -> [w341 w641]
      tunnel: w330 -> [w340 w640]
      tunnel: [w339 w640] -> w329
      frame No Error {
        n192 = case shown="\"Donate\"" w344 {
          tunnel: w343 -> [w347 w354 w377 w386 _ _ _ w486 w501 w513 _ w522 w525 _ w555 _ _ w612 _ _ _]
          tunnel: [_ w352 w376 w384 _ _ _ w486 w499 w512 _ w522 w525 _ _ _ _ w609 _ _ _] -> w342
          tunnel: w341 -> [w349 w351 w381 w383 w395 w469 w485 w492 w506 w516 w518 w521 w524 w531 w560 w587 w608 w616 w621 w626 w631]
          tunnel: w340 -> [w348 w350 w370 w382 w394 w468 w483 w488 w495 w515 w519 w520 w523 w527 w557 w585 w604 w611 w620 w625 w628]
          tunnel: [w345 w350 w370 w382 w393 w468 w482 w487 w496 w509 w519 w520 w523 w526 w556 w584 w601 w610 w617 w624 w627] -> w339
          tunnel: [w349 w351 w381 w383 w395 w469 w485 w492 w506 w516 w518 w521 w524 w531 w560 w587 w608 w616 w621 w626 w631] -> w338
          frame "Save Portfolio", Default {
            n193 = property on="Current Portfolio Path" class="Chm"() -> ("Value"=w346:path)  [unwired: 2 in, 2 out]
            n194 = call "Save_Portfolio.vi"("error in (no error)"=w347, "path"=w346, "Portfolio in"=w348) -> ("Portfolio en sortie"=w345:refnum<class "Portfolio.lvclass">)  [unwired: 7 in, 1 out]
          }
          frame "Test Progress Bar" {
            w357 = TRUE ("Go")
            w361 = 100.0 ("y")
            n195 = call "Update UI User Notification.vi"("Cancel Visibile? (F)"=w357, "Progress Bar Visibile? (F)"=w357, "Error In"=w354, "Busy Cursor? (F)"=w357) -> ("Error Out"=w356:errorcluster)  [unwired: 6 in, 1 out]
            n196 = Divide(x=30000.0 ("y"), y=w361) -> (x/y=w360:dbl)
            n197 = for {
              N: w361 -> [_]
              tunnel: w360 -> [w369]
              tunnel: ["Cancel"] -> w359
              shift-right: [w363] -> w355
              shift-left: w356 -> [w364]
              i -> [w367]
              stop <- "Cancel" stop-if-true
              w366 = TRUE ("Go")
              n198 = Wait (ms)(milliseconds to wait=w369) -> ()  [unwired: 1 out]
              n199 = call "Update UI User Notification.vi"("Progress Bar Value (0)"=w367, "Cancel Visibile? (F)"=w366, "Progress Bar Visibile? (F)"=w366, "Error In"=w364, "Busy Cursor? (F)"=w366, "Status Bar (\"\")"="Saving..." ("Status Bar Text 2")) -> ("Error Out"=w363:errorcluster)  [unwired: 4 in, 1 out]
            }
            n200 = case shown="Vrai" w359 {
              tunnel: "Save Cancelled" ("Status Bar Text 2") -> [_ w362]
              frame False {
              }
              frame True {
                n201 = One Button Dialog(message=w362) -> ()  [unwired: 1 in, 1 out]
              }
            }
            n202 = call "Update UI User Notification.vi"("Error In"=w355) -> ("Error Out"=w352:errorcluster)  [unwired: 9 in, 1 out]
          }
          frame "Panel Resize" {
            n203 = property on="Left Menu Pane" class="Pann"(error in=w377) -> (error out=w378:errorcluster, "Height"=w375:u32)  [unwired: 1 in, 1 out]
            n204 = Divide(x=w375, y=u32 2) -> (x/y=w373:dbl)
            n205 = Subtract(x=w373, y=u32 100) -> (x-y=w371:dbl)
            n206 = property on="Collapse Left" class="Bool (strict)"("Top"=w371) -> ()  [unwired: 2 in, 2 out]
            n207 = property on="Collapse Right" class="Bool (strict)"("Top"=w371) -> ()  [unwired: 2 in, 2 out]
            n208 = Subtract(x=w375, y=u32 30) -> (x-y=w379:u32)
            n209 = property on="Help" class="Bool"(error in=w378, "Top"=w379) -> (error out=w376:errorcluster)  [unwired: 1 in, 1 out]
          }
          frame "Acquire" {
            n210 = call "Simulate Signal"("error in (no error)"=w386) -> ("Sine with Uniform Noise"=w392:dynamicdata, "error out"=w387:errorcluster)  [unwired: 13 in]
            n211 = call "Mask and Limit Testing"("error in"=w387, "Signals"=w392) -> ("error out"=w385:errorcluster, "Point Evaluation"=w388:dynamicdata)  [unwired: 6 in, 2 out]
            n212 = control-ref of="Table Control"() -> (w390:refnum<vi>)
            n213 = call "Convert from Dynamic Data"("Dynamic Data Type"=w388) -> ("Array"=w389:bool[])  [unwired: 3 in]
            n214 = call "Format Data into Table.vi"("error in (no error)"=w385, "Passed?"=w389, "Signals"=w392, "Tbl Refnum"=w390) -> ("error out"=w384:errorcluster, "Table"=→"Table Control":string[][])  [unwired: 5 in, 1 out]
          }
          frame "Calc" {
            n215 = stacked-sequence {
              seq-local: [_ w407 _ _ _ _ _ _] -> [_ _ w425 _ _ _ _ _]
              seq-local: [_ w405 _ _ _ _ _ _] -> [_ _ _ w436 w442 _ w454 w460]
              seq-local: [_ w397 _ _ _ _ _ _] -> [_ _ _ _ _ w448 _ _]
              tunnel: w394 -> [_ w415 w435 _ _ _ _ _]
              tunnel: [_ w412 _ _ _ _ _ _] -> w393
              frame #0 {
                n216 = property on="calc Done ?" class="Bool (strict)"("Value"=FALSE ("calc Done ?")) -> ()  [unwired: 2 in, 2 out]
              }
              frame #1 {
                w402 = TRUE ("Go")
                w399 = 100.0 ("y")
                n217 = Get Date/Time In Seconds() -> (seconds since 1Jan1904=w414:timestamp)
                n218 = call "Calc_Portfolio_at_Date.vi"("Portfolio en entrée"=w415, "Date"=w414) -> ("Change-couleurs"=w397:u32[], "Portfolio en sortie"=w413:refnum<class "Portfolio.lvclass">, "Valo-couleurs"=w405:u32[], "Montant investi"=w407:dbl, "Done ?"=→"calc Done ?":bool, "Tableau"=w406:string[][])  [unwired: 5 in, 3 out]
                n219 = call "Lire Parameters.vi"("Portfolio en entrée"=w413) -> ("Parameters"=w411:T12, "Portfolio en sortie"=w412:refnum<class "Portfolio.lvclass">)  [unwired: 9 in]
                n220 = call "Update UI User Notification.vi"("Cancel Visibile? (F)"=w402, "Progress Bar Visibile? (F)"=w402, "Busy Cursor? (F)"=w402) -> ("Error Out"=w403:errorcluster)  [unwired: 7 in, 1 out]
                n221 = Divide(x=3000.0 ("y"), y=w399) -> (x/y=w400:dbl)
                n222 = for {
                  N: w399 -> [_]
                  tunnel: w400 -> [w422]
                  shift-right: [w417] -> w404
                  shift-left: w403 -> [w418]
                  i -> [w421]
                  stop <- w416 stop-if-true
                  w420 = TRUE ("Go")
                  n223 = Wait (ms)(milliseconds to wait=w422) -> ()  [unwired: 1 out]
                  n224 = property on="calc Done ?" class="Bool (strict)"() -> ("Value"=w416:bool)  [unwired: 2 in, 2 out]
                  n225 = call "Update UI User Notification.vi"("Progress Bar Value (0)"=w421, "Cancel Visibile? (F)"=w420, "Progress Bar Visibile? (F)"=w420, "Error In"=w418, "Busy Cursor? (F)"=w420, "Status Bar (\"\")"="Mise a jour..." ("Status Bar Text 2")) -> ("Error Out"=w417:errorcluster)  [unwired: 4 in, 1 out]
                }
                n226 = Unbundle By Name(w411) -> ("Cash"=→"Solde espèces :":dbl, "Total"=→"Evaluation totale :":dbl, "Investissements"=→"Investissement total :":dbl)
                n227 = property on="Portefeuille" class="ListeMCol (strict)"("ItemNames"=w406) -> ()  [unwired: 2 in, 2 out]
                n228 = call "Update UI User Notification.vi"("Error In"=w404) -> ()  [unwired: 9 in, 2 out]
              }
              frame #2 {
                n229 = call "Lire Parameters.vi"("Portfolio en entrée"=w435) -> ("Parameters"=w434:T12)  [unwired: 9 in, 1 out]
                n230 = Unbundle By Name(w434) -> ("Performance sur 1 an (en %)"=→"Performance sur 1an :":dbl, "Performance Totale (en %)"=→"Performance Totale :":dbl, "Cash"=w429:dbl, "Total"=w424:dbl)
                n231 = Divide(x=w425, y=w424) -> (x/y=w426:dbl)
                n232 = Divide(x=w429, y=w424) -> (x/y=w432:dbl)
                n233 = Multiply(x=w426, y=100.0) -> (x*y=→"% investi":dbl)
                n234 = Multiply(x=w432, y=100.0) -> (x*y=→"% cash":dbl)
                "Montant investi :" <- w425
              }
              frame #3 {
                n235 = for {
                  tunnel: w436 -> [w438] mode=indexing
                  i -> [w437]
                  n236 = Bundle By Name(cluster=T10 {"Row"=0, "Column"=0} ("Cellule active : cellule active"), "Row"=w437, "Column"=5) -> (w440:T10)
                  n237 = property on="Portefeuille" class="ListeMCol (strict)"("ActiveCell"=w440, "CellFontColor"=w438) -> ()  [unwired: 2 in, 2 out]
                }
              }
              frame #4 {
                n238 = for {
                  tunnel: w442 -> [w444] mode=indexing
                  i -> [w443]
                  n239 = Bundle By Name(cluster=T10 {"Row"=0, "Column"=0} ("Cellule active : cellule active"), "Row"=w443, "Column"=6) -> (w446:T10)
                  n240 = property on="Portefeuille" class="ListeMCol (strict)"("ActiveCell"=w446, "CellFontColor"=w444) -> ()  [unwired: 2 in, 2 out]
                }
              }
              frame #5 {
                n241 = for {
                  tunnel: w448 -> [w450] mode=indexing
                  i -> [w449]
                  n242 = Bundle By Name(cluster=T10 {"Row"=0, "Column"=0} ("Cellule active : cellule active"), "Row"=w449, "Column"=7) -> (w452:T10)
                  n243 = property on="Portefeuille" class="ListeMCol (strict)"("ActiveCell"=w452, "CellFontColor"=w450) -> ()  [unwired: 2 in, 2 out]
                }
              }
              frame #6 {
                n244 = for {
                  tunnel: w454 -> [_] mode=indexing
                  i -> [w456]
                  n245 = Bundle By Name(cluster=T10 {"Row"=0, "Column"=0} ("Cellule active : cellule active"), "Row"=w456, "Column"=0) -> (w458:T10)
                  n246 = property on="Portefeuille" class="ListeMCol (strict)"("ActiveCell"=w458, "CellFontColor"=u32 0 ("Color")) -> ()  [unwired: 2 in, 2 out]
                }
              }
              frame #7 {
                n247 = for {
                  tunnel: w460 -> [_] mode=indexing
                  i -> [w462]
                  n248 = Bundle By Name(cluster=T10 {"Row"=0, "Column"=0} ("Cellule active : cellule active"), "Row"=w462, "Column"=1) -> (w464:T10)
                  n249 = property on="Portefeuille" class="ListeMCol (strict)"("ActiveCell"=w464, "CellFontColor"=u32 0 ("Color")) -> ()  [unwired: 2 in, 2 out]
                }
              }
            }
          }
          frame "Display tarif" {
            n250 = property on="Provider" class="Énum (strict)"() -> ("Strings []"=w467:string[])  [unwired: 2 in, 2 out]
            n251 = for {
              tunnel: w467 -> [w471] mode=indexing
              tunnel: [w473] -> w466 mode=indexing
              i -> [w470]
              n252 = call "Calcul Tarifs Bourse.vi"("Provider"=w470) -> ("Graphe"=w474:dbl[])  [unwired: 10 in]
              n253 = Bundle By Name(cluster=waveform(dbl) {"t0"=timestamp(0 s since 1904-01-01), "dt"=1.0, "Y"=[]} ("waveform"), "Y"=w474) -> (w473:waveform(dbl))
              n254 = property on="Tarifs" class="GraphWF (strict)"("Active Plot"=w470) -> (error out=w472:errorcluster)  [unwired: 2 in, 1 out]
              n255 = property on="Tarifs" class="GraphWF (strict)"(error in=w472, "Plot.Plot Name"=w471) -> ()  [unwired: 1 in, 2 out]
            }
            "Tarifs" <- w466
          }
          frame "Calc History" {
            n256 = Get Date/Time In Seconds() -> (seconds since 1Jan1904=w484:timestamp)
            n257 = call "Calc_Portfolio_History_at_Date.vi"("Portfolio en entrée"=w483, "Date"=w484) -> ("Portfolio en sortie"=w482:refnum<class "Portfolio.lvclass">, "Hist Valeur PF"=w479:dbl[], "Hist Taux de Perf"=w476:dbl[])  [unwired: 9 in, 2 out]
            n258 = Bundle By Name("Y"=w479) -> (w478:waveform(dbl))  [unwired: 1 in]
            n259 = Bundle By Name("Y"=w476) -> (w477:waveform(dbl))  [unwired: 1 in]
            n260 = Insert Into Array(array=waveform(dbl)[] [] ("waveform array"), new element #1=w478, new element #2=w477) -> (→"Waveform Graph":waveform(dbl)[])  [unwired: 1 in]
          }
          frame "New Portfolio" {
            n261 = property on="Config File Path" class="Chm"() -> ("Value"=w491:path)  [unwired: 2 in, 2 out]
            n262 = call "Dlg-New-Portfolio.vi"("Config File Path"=w491) -> ("Canceled"=w490:bool, "Portfolio out"=w489:refnum<class "Portfolio.lvclass">)  [unwired: 8 in, 1 out]
            n263 = case shown="Vrai" w490 {
              tunnel: w489 -> [w493 _]
              tunnel: w488 -> [_ w494]
              tunnel: [w493 w494] -> w487
              frame False {
              }
              frame True {
              }
            }
          }
          frame "Open Portfolio" {
            n264 = call "Boîte de dialogue de fichier"("error in"=w501, "pattern (all files)"="*.xlp", "pattern label"="XLP") -> ("selected path"=w502:path, "cancelled"=w498:bool, "error out"=w500:errorcluster)  [unwired: 9 in, 1 out]
            n265 = property on="Config File Path" class="Chm"() -> ("Value"=w505:path)  [unwired: 2 in, 2 out]
            n266 = call "Load_Portfolio.vi"("Config File path"=w505, "error in (no error)"=w500, "path"=w502) -> ("error out"=w499:errorcluster, "Portfolio en sortie"=w497:refnum<class "Portfolio.lvclass">)  [unwired: 7 in]
            n267 = case shown="Vrai" w498 {
              tunnel: w497 -> [w507 _]
              tunnel: [w507 w508] -> w496
              tunnel: w495 -> [_ w508]
              frame False {
              }
              frame True {
              }
            }
          }
          frame "Add Operation" {
            n268 = call "Lire Operations.vi"("Portfolio en entrée"=w515) -> ("Operations.lvclass"=w514:refnum<class "Operations.lvclass">, "Portfolio en sortie"=w510:refnum<class "Portfolio.lvclass">)  [unwired: 9 in]
            n269 = call "Dlg-Add-Operation.vi"("error in (no error)"=w513, "Operations in"=w514) -> ("error out"=w512:errorcluster, "Operations out"=w511:refnum<class "Operations.lvclass">)  [unwired: 7 in, 1 out]
            n270 = call "Écrire Operations.vi"("Operations.lvclass"=w511, "Portfolio en entrée"=w510) -> ("Portfolio en sortie"=w509:refnum<class "Portfolio.lvclass">)  [unwired: 9 in]
          }
          frame "Donate" {
            n271 = call "open_browser_send_url.vi"("Enter a URL and run the VI"="https://www.paypal.com/cgi-bin/webscr?cmd=_s-xclick&hosted_button_id=Z47KKFPK87JBG") -> ()  [unwired: 1 in]
          }
          frame "Print" {
            # "Put your printing code here."
            n272 = Unbundle By Name(w521) -> ()  [unwired: 2 out]
          }
          frame "Help" {
          }
          frame "Edit Operation" {
            n273 = property on="Operations" class="ListeMCol (strict)"() -> ("Value"=w530:i32[])  [unwired: 2 in, 2 out]
            n274 = Index Array(array=w530) -> (element=w528:i32)  [unwired: 1 in]
            n275 = Greater Or Equal To 0?(x=w528) -> (x >= 0?=w529:bool)
            n276 = case shown="Vrai" w529 {
              tunnel: w528 -> [_ w533]
              tunnel: w527 -> [w532 w540]
              tunnel: [w532 w536] -> w526
              frame False {
              }
              frame True {
                n277 = call "Lire Operations.vi"("Portfolio en entrée"=w540) -> ("Operations.lvclass"=w539:refnum<class "Operations.lvclass">, "Portfolio en sortie"=w537:refnum<class "Portfolio.lvclass">)  [unwired: 9 in]
                n278 = call "Find Operations.vi"("Position"=w533, "Operations en entrée"=w539) -> ("found?"=w538:bool, "Parameters"=w535:T13, "Operations en sortie"=w534:refnum<class "Operations.lvclass">)  [unwired: 6 in, 1 out]
                n279 = case shown="Vrai" w538 {
                  tunnel: w537 -> [w542 w547]
                  tunnel: [w542 w545] -> w536
                  tunnel: w535 -> [_ w543]
                  tunnel: w533 -> [_ w549]
                  tunnel: w534 -> [_ w548]
                  frame False {
                    n280 = property on="Edit OP" class="Bool"("DisabledEnum"=T8."Disabled and Grayed Out" ("Désactivé")) -> ()  [unwired: 2 in, 2 out]
                  }
                  frame True {
                    n281 = call "Dlg-Edit-Operation.vi"("Parameters"=w543, "Key"=w549, "Operations in"=w548) -> ("Canceled"=w544:bool, "Operations out"=w546:refnum<class "Operations.lvclass">)  [unwired: 6 in, 1 out]
                    n282 = case shown="Faux" w544 {
                      tunnel: w547 -> [w552 w553]
                      tunnel: w546 -> [w551 _]
                      tunnel: [w550 w553] -> w545
                      frame False {
                        n283 = call "Écrire Operations.vi"("Operations.lvclass"=w551, "Portfolio en entrée"=w552) -> ("Portfolio en sortie"=w550:refnum<class "Portfolio.lvclass">)  [unwired: 9 in]
                      }
                      frame True {
                      }
                    }
                  }
                }
              }
            }
          }
          frame "Edit Exchange" {
            n284 = property on="Exchanges" class="ListeMCol (strict)"(error in=w555) -> ("Value"=w554:i32[])  [unwired: 1 in, 2 out]
            n285 = Index Array(array=w554) -> (element=w558:i32)  [unwired: 1 in]
            n286 = Greater Or Equal To 0?(x=w558) -> (x >= 0?=w559:bool)
            n287 = case shown="Vrai" w559 {
              tunnel: w558 -> [_ w562]
              tunnel: w557 -> [w561 w569]
              tunnel: [w561 w565] -> w556
              frame False {
              }
              frame True {
                n288 = call "Lire Exchanges.vi"("Portfolio en entrée"=w569) -> ("Exchanges.lvclass"=w568:refnum<class "Exchanges.lvclass">, "Portfolio en sortie"=w566:refnum<class "Portfolio.lvclass">)  [unwired: 9 in]
                n289 = call "Find Exchanges.vi"("Position"=w562, "Exchanges en entrée"=w568) -> ("Parameters"=w564:T16, "found?"=w567:bool, "Exchanges en sortie"=w563:refnum<class "Exchanges.lvclass">)  [unwired: 6 in, 1 out]
                n290 = case shown="Vrai" w567 {
                  tunnel: w566 -> [w571 w576]
                  tunnel: [w571 w574] -> w565
                  tunnel: w564 -> [_ w572]
                  tunnel: w562 -> [_ w578]
                  tunnel: w563 -> [_ w577]
                  frame False {
                    n291 = property on="Edit Exch" class="Bool"("DisabledEnum"=T8."Disabled and Grayed Out" ("Désactivé")) -> ()  [unwired: 2 in, 2 out]
                  }
                  frame True {
                    n292 = call "Dlg-Edit-Exchanges.vi"("Parameters"=w572, "Key"=w578, "Exchanges in"=w577) -> ("Canceled"=w573:bool, "Exchanges out"=w575:refnum<class "Exchanges.lvclass">)  [unwired: 6 in, 1 out]
                    n293 = case shown="Faux" w573 {
                      tunnel: w576 -> [w581 w582]
                      tunnel: w575 -> [w580 _]
                      tunnel: [w579 w582] -> w574
                      frame False {
                        n294 = call "Écrire Exchanges.vi"("Exchanges.lvclass"=w580, "Portfolio en entrée"=w581) -> ("Portfolio en sortie"=w579:refnum<class "Portfolio.lvclass">)  [unwired: 9 in]
                      }
                      frame True {
                      }
                    }
                  }
                }
              }
            }
          }
          frame "Delete Operation" {
            n295 = Two Button Dialog(message="Etes-vous Sûr ?") -> (T button?=w586:bool)  [unwired: 2 in]
            n296 = case shown="Vrai" w586 {
              tunnel: w585 -> [w588 w594]
              tunnel: [w588 w589] -> w584
              frame False {
              }
              frame True {
                n297 = property on="Operations" class="ListeMCol (strict)"() -> ("Value"=w595:i32[])  [unwired: 2 in, 2 out]
                n298 = call "Lire Operations.vi"("Portfolio en entrée"=w594) -> ("Operations.lvclass"=w593:refnum<class "Operations.lvclass">, "Portfolio en sortie"=w590:refnum<class "Portfolio.lvclass">)  [unwired: 9 in]
                n299 = Index Array(array=w595) -> (element=w592:i32)  [unwired: 1 in]
                n300 = call "Delete Operations.vi"("Position"=w592, "Operations en entrée"=w593) -> ("Operations en sortie"=w591:refnum<class "Operations.lvclass">)  [unwired: 8 in, 1 out]
                n301 = call "Écrire Operations.vi"("Operations.lvclass"=w591, "Portfolio en entrée"=w590) -> ("Portfolio en sortie"=w589:refnum<class "Portfolio.lvclass">)  [unwired: 9 in]
              }
            }
          }
          frame "Update PFLine ToolStrip" {
            n302 = property on="Portefeuille" class="ListeMCol (strict)"() -> ("ItemNames"=w607:string[][])  [unwired: 2 in, 2 out]
            n303 = property on="Portefeuille" class="ListeMCol (strict)"() -> ("Value"=w606:i32)  [unwired: 2 in, 2 out]
            n304 = Index Array(array=w607, index (row)=w606, index (col)=0 ("indice désactivé (col)")) -> (element=w603:string)
            n305 = call "Find_Exchanges.vi"("Type"=Find_Exchanges."Find_From_Label", "To_be_Found"=w603, "Portfolio en entrée"=w604) -> ("Gain/loss"=w598:dbl, "Portfolio en sortie"=w601:refnum<class "Portfolio.lvclass">)  [unwired: 5 in, 2 out]
            n306 = Format Into String(format string="%.2f" ("chaîne de format"), w598) -> (resulting string=w597:string)  [unwired: 2 in, 1 out]
            n307 = Concatenate Strings("Gain / Perte totale sur cette ligne : " ("Info-bulle"), w597) -> (w596:string)
            n308 = call "Update UI User Notification.vi"("Status Bar (\"\")"=w596) -> ()  [unwired: 9 in, 2 out]
            n309 = property on="Portefeuille" class="ListeMCol (strict)"("TipStrip"=w596) -> ()  [unwired: 2 in, 2 out]
          }
          frame "Add Exchange" {
            n310 = call "Lire Exchanges.vi"("Portfolio en entrée"=w611) -> ("Exchanges.lvclass"=w615:refnum<class "Exchanges.lvclass">, "Portfolio en sortie"=w613:refnum<class "Portfolio.lvclass">)  [unwired: 9 in]
            n311 = call "Dlg-Add-Exchanges.vi"("error in (no error)"=w612, "Exchanges in"=w615) -> ("error out"=w609:errorcluster, "Exchanges out"=w614:refnum<class "Exchanges.lvclass">)  [unwired: 7 in, 1 out]
            n312 = call "Écrire Exchanges.vi"("Exchanges.lvclass"=w614, "Portfolio en entrée"=w613) -> ("Portfolio en sortie"=w610:refnum<class "Portfolio.lvclass">)  [unwired: 9 in]
          }
          frame "Update Operations" {
            n313 = call "Lire Operations.vi"("Portfolio en entrée"=w620) -> ("Operations.lvclass"=w619:refnum<class "Operations.lvclass">, "Portfolio en sortie"=w617:refnum<class "Portfolio.lvclass">)  [unwired: 9 in]
            n314 = call "Get All Operations.vi"("Operations en entrée"=w619) -> ("tableau a afficher"=w618:string[][])  [unwired: 6 in, 4 out]
            n315 = property on="Operations" class="ListeMCol (strict)"("ItemNames"=w618) -> ()  [unwired: 2 in, 2 out]
          }
          frame "Update Exchanges" {
            n316 = call "Lire Exchanges.vi"("Portfolio en entrée"=w625) -> ("Exchanges.lvclass"=w623:refnum<class "Exchanges.lvclass">, "Portfolio en sortie"=w624:refnum<class "Portfolio.lvclass">)  [unwired: 9 in]
            n317 = call "Get All Exchanges.vi"("Exchanges en entrée"=w623) -> ("tableau a afficher"=w622:string[][])  [unwired: 6 in, 4 out]
            n318 = property on="Exchanges" class="ListeMCol (strict)"("ItemNames"=w622) -> ()  [unwired: 2 in, 2 out]
          }
          frame "Delete Exchange" {
            n319 = Two Button Dialog(message="Etes-vous Sûr ?") -> (T button?=w630:bool)  [unwired: 2 in]
            n320 = case shown="Vrai" w630 {
              tunnel: w628 -> [w632 w639]
              tunnel: [w632 w634] -> w627
              frame False {
              }
              frame True {
                n321 = property on="Exchanges" class="ListeMCol (strict)"() -> ("Value"=w633:i32[])  [unwired: 2 in, 2 out]
                n322 = call "Lire Exchanges.vi"("Portfolio en entrée"=w639) -> ("Exchanges.lvclass"=w638:refnum<class "Exchanges.lvclass">, "Portfolio en sortie"=w635:refnum<class "Portfolio.lvclass">)  [unwired: 9 in]
                n323 = Index Array(array=w633) -> (element=w637:i32)  [unwired: 1 in]
                n324 = call "Delete Exchanges.vi"("Position"=w637, "Exchanges en entrée"=w638) -> ("Exchanges en sortie"=w636:refnum<class "Exchanges.lvclass">)  [unwired: 8 in, 1 out]
                n325 = call "Écrire Exchanges.vi"("Exchanges.lvclass"=w636, "Portfolio en entrée"=w635) -> ("Portfolio en sortie"=w634:refnum<class "Portfolio.lvclass">)  [unwired: 9 in]
              }
            }
          }
        }
      }
      frame Error {
      }
    }
  }
  n326 = Release Queue(queue=w6) -> ()  [unwired: 2 in, 3 out]
